vi "time_arrive.vi"() -> ()   [LabVIEW 2017]
panel:
  out "输出数组":dbl[][](array[numeric])
  in  "数组 4":dbl[][](array[numeric])
  in  "数组 3":dbl[][](array[numeric])
  out "添加的数组":string[][][](array[string])
  out "数组 2":i32[](array[numeric])
  out "交织的数组":string[](array[string])
  out "大小":i32
  in  "数组":string[](array[string])
  out "保存名":string
  out "数据保存路径":path
  out "字符串":string
  in  "恒温结束分钟":dbl
  in  "恒温结束小时":dbl
  out "时间到":bool
  in  "分钟":dbl
  in  "小时":dbl
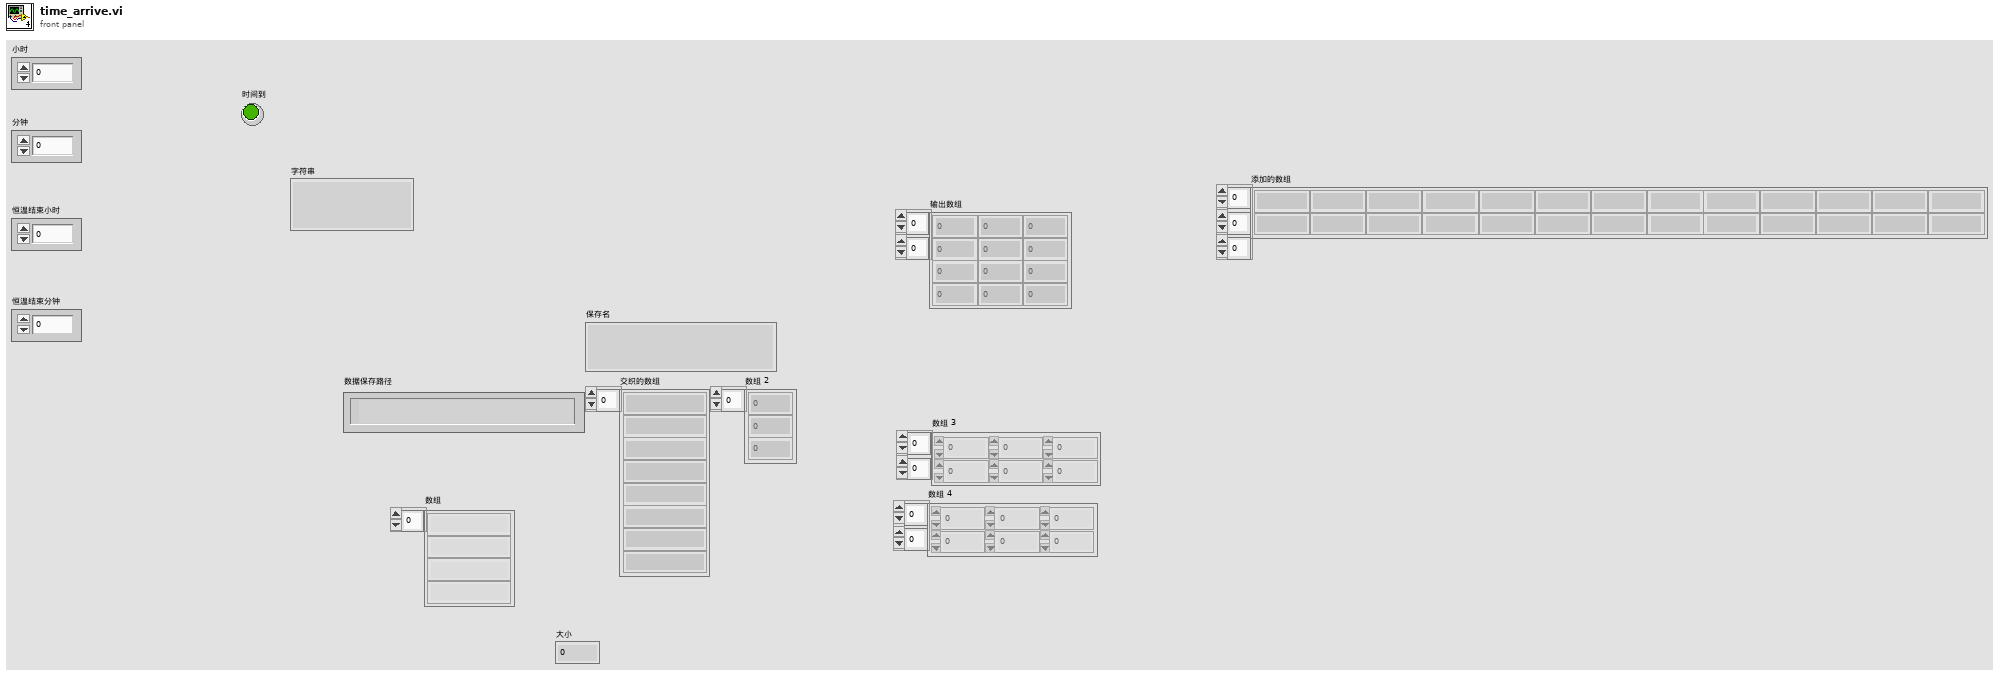
[diagram p1: front panel]
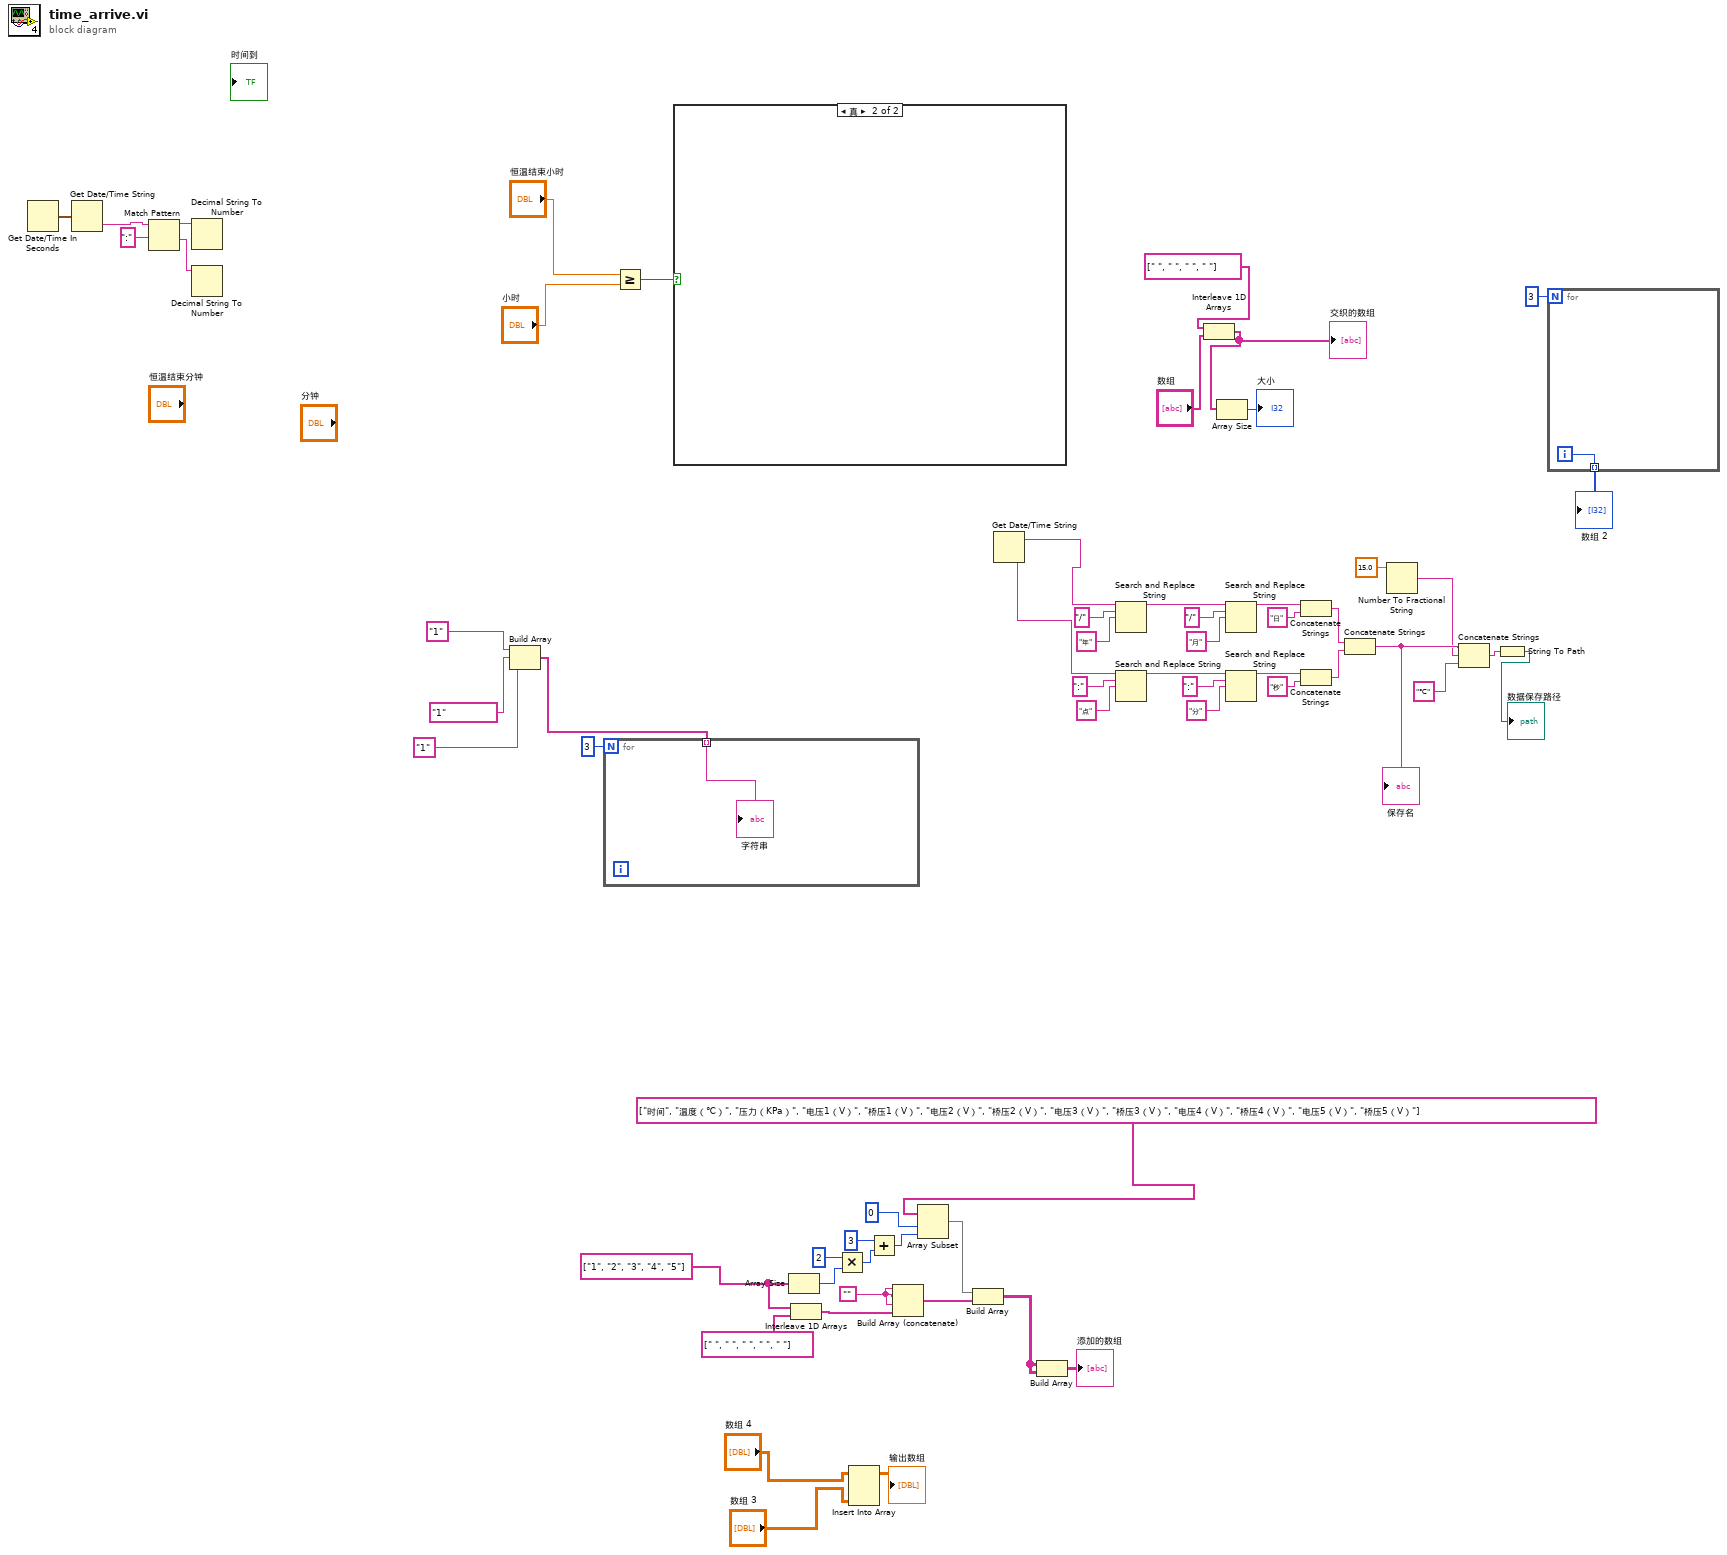
[diagram p0: block diagram]
diagram:
  w7 = string[] ["1", "2", "3", "4", "5"]
  w11 = ""
  n1 = Get Date/Time In Seconds() -> (seconds since 1Jan1904=w61:timestamp)
  n2 = Get Date/Time String(seconds (now)=w61) -> (time string=w57:string)  [unwired: 2 in, 1 out]
  n3 = Match Pattern(string=w57, regular expression=":" ("正则表达式")) -> (before substring=w60:string, after substring=w59:string)  [unwired: 1 in, 2 out]
  n4 = Decimal String To Number(string=w60) -> ()  [unwired: 2 in, 2 out]
  n5 = Decimal String To Number(string=w59) -> ()  [unwired: 2 in, 2 out]
  n6 = Build Array("1", "1", "1") -> (w49:string[])
  n7 = for {
    N: 3 -> [_]
    tunnel: w49 -> [w62] mode=indexing
    "字符串" <- w62
  }
  n8 = Greater Or Equal?(x="恒温结束小时", y="小时") -> (x >= y?=w54:bool)
  n9 = case shown="真" w54 {
    frame False {
    }
    frame True {
    }
  }
  n10 = Array Size(array=w7) -> (size(s)=w18:i32)
  n11 = Interleave 1D Arrays(w7, string[] [" ", " ", " ", " ", " "]) -> (w12:string[])
  n12 = Multiply(x=2, y=w18) -> (x*y=w14:i32)
  n13 = Insert Into Array(array="数组 4", new element="数组 3") -> (→"输出数组":dbl[][])  [unwired: 2 in]
  n14 = Add(x=3, y=w14) -> (x+y=w13:i32)
  n15 = Build Array (concatenate)(w11, w11, w11, w12) -> (w9:string[])
  n16 = Array Subset(array=string[] ["时间", "温度（℃）", "压力（KPa）", "电压1（V）", "桥压1（V）", "电压2（V）", "桥压2（V）", "电压3（V）", "桥压3（V）", "电压4（V）", "桥压4（V）", "电压5（V）", "桥压5（V）"], index=0 ("索引"), length=w13) -> (w10:string[])
  n17 = Build Array(w10, w9) -> (w5:string[][])
  n18 = Get Date/Time String() -> (date string=w31:string, time string=w30:string)  [unwired: 3 in]
  n19 = Build Array(w5, w5) -> (→"添加的数组":string[][][])
  n20 = Search and Replace String(input string=w31, search string="/" ("搜索字符串"), replace string="年" ("替换字符串(\"\")")) -> (result string=w46:string)  [unwired: 5 in, 3 out]
  n21 = Search and Replace String(input string=w30, search string=":" ("搜索字符串"), replace string="点" ("替换字符串(\"\")")) -> (result string=w40:string)  [unwired: 5 in, 3 out]
  n22 = Interleave 1D Arrays(string[] [" ", " ", " ", " "], "数组") -> (w21:string[])
  "交织的数组" <- w21
  n23 = Array Size(array=w21) -> (size(s)=→"大小":i32)
  n24 = Search and Replace String(input string=w46, search string="/" ("搜索字符串"), replace string="月" ("替换字符串(\"\")")) -> (result string=w43:string)  [unwired: 5 in, 3 out]
  n25 = Search and Replace String(input string=w40, search string=":" ("搜索字符串"), replace string="分" ("替换字符串(\"\")")) -> (result string=w36:string)  [unwired: 5 in, 3 out]
  n26 = Concatenate Strings(w43, "日" ("字符串")) -> (w33:string)
  n27 = Concatenate Strings(w36, "秒" ("字符串")) -> (w34:string)
  n28 = Concatenate Strings(w33, w34) -> (w29:string)
  "保存名" <- w29
  n29 = Number To Fractional String(number=15.0 ("数字")) -> (F-format string=w28:string)  [unwired: 3 in]
  n30 = Concatenate Strings(w29, w28, "℃" ("字符串")) -> (w32:string)
  n31 = String To Path(string=w32) -> (path=→"数据保存路径":path)
  n32 = for {
    N: 3 -> [_]
    tunnel: [w63] -> w19 mode=indexing
    i -> [w63]
  }
  "数组 2" <- w19
